vi "Channel Selection.vi"(8 "error in (no error)":errorcluster, 10 "NIVS.System Definition Root":refnum<k24>, 11 "Input":T1) -> (0 "error out":errorcluster, 3 "Output":T1)   [LabVIEW 2010]
uses:
  Data Typedef.ctl
  NationalInstruments.VeriStand.SystemStorage
panel:
  out "Full Channel Path":string
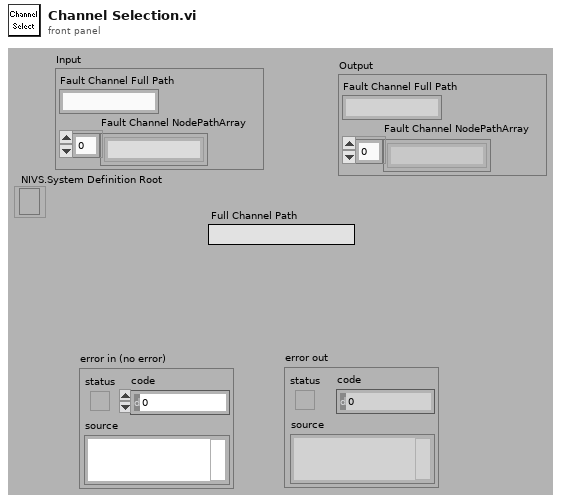
[diagram p1: front panel]
types:
  T1 = typedef "Data Typedef.ctl" = cluster{"Fault Channel Full Path":string, "Fault Channel NodePathArray":string[]}
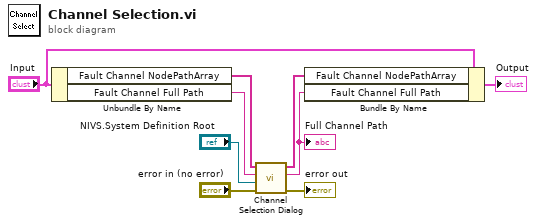
[diagram p0: block diagram]
diagram:
  n1 = Unbundle By Name("Input") -> ("Fault Channel NodePathArray"=w1:string[], "Fault Channel Full Path"=w2:string)
  n2 = call "Channel Selection Dialog.vi"("error in (no error)"="error in (no error)", "NIVS.System Definition Root"="NIVS.System Definition Root", "NodePath"=w2, "NodePathArray"=w1) -> ("error out"=→"error out":errorcluster, "Selected NodePath"=w8:string, "Selected NodePathArray"=w4:string[])  [unwired: 5 in]
  "Full Channel Path" <- w8
  n3 = Bundle By Name(cluster="Input", "Fault Channel NodePathArray"=w4, "Fault Channel Full Path"=w8) -> (→"Output":T1)
